vi "IsEnumOrEnumArrayControl.vi"(8 "error in (no error)":errorcluster, 11 "Control reference in":refnum<vi>) -> (0 "error out":errorcluster, 2 "IsEnumOrEnumArrayControl":bool, 3 "Control reference out":refnum<vi>)   [LabVIEW 2020, in "MeasurementLink Measurement Server.lvlib"]
uses:
  MeasurementLink Measurement Server.lvlib
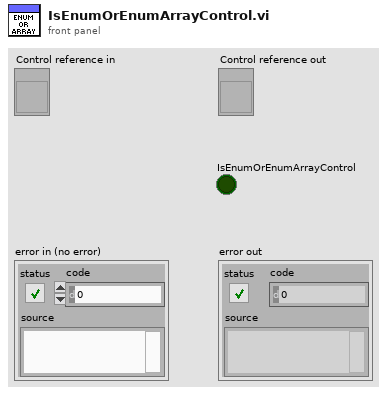
[diagram p1: front panel]
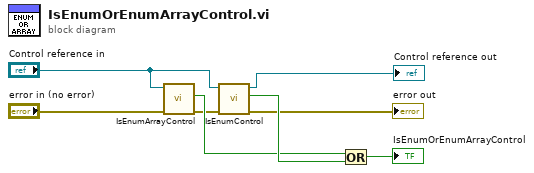
[diagram p0: block diagram]
diagram:
  n1 = call "IsEnumArrayControl.vi"("error in (no error)"="error in (no error)", "Control reference in"="Control reference in") -> ("error out"=w4:errorcluster, "IsEnumArrayControl"=w6:bool)  [unwired: 7 in, 1 out]
  n2 = call "IsEnumControl.vi"("error in (no error)"=w4, "Control reference in"="Control reference in") -> ("error out"=→"error out":errorcluster, "IsEnumControl"=w7:bool, "Control reference out"=→"Control reference out":refnum<vi>)  [unwired: 7 in]
  n3 = Or(x=w6, y=w7) -> (x .or. y?=→"IsEnumOrEnumArrayControl":bool)
